vi "Camera_with_init.vi"(0 "Frames":T1=1, 5 "IntegrationTime (us)":dbl=1.0 min=0.1 max=5000.0 step=0.1, 9 "Frame Size (Row x Col)":u16(ring) items=["128x128", "96x128", "64x128", "32x128"], 11 "Timeout":i32) -> (6 "TempK":dbl, 8 "FrameData even":dbl[][][](array[numeric]), 15 "FrameData odd":dbl[][][](array[numeric]))   [LabVIEW 2020]
uses:
  Control 1.ctl
panel:
  out "subarray":dbl[][](array[numeric])
  out "Delta T":dbl[][](array[numeric])
  out "FrameData":dbl[][][](array[numeric])
  out "ExtChData":dbl[][](array[numeric])
  in  "ExChs":i32
  in  "Acq Trigger?":bool
  in  "Offset":i32=128 min=0 max=255 step=1
  out "Actual (us)":dbl
  out "MaxFrameRate":dbl
  out "First Image":dbl[][](graph)
  out "error":errorcluster
  # "IMAGE SETTINGS"
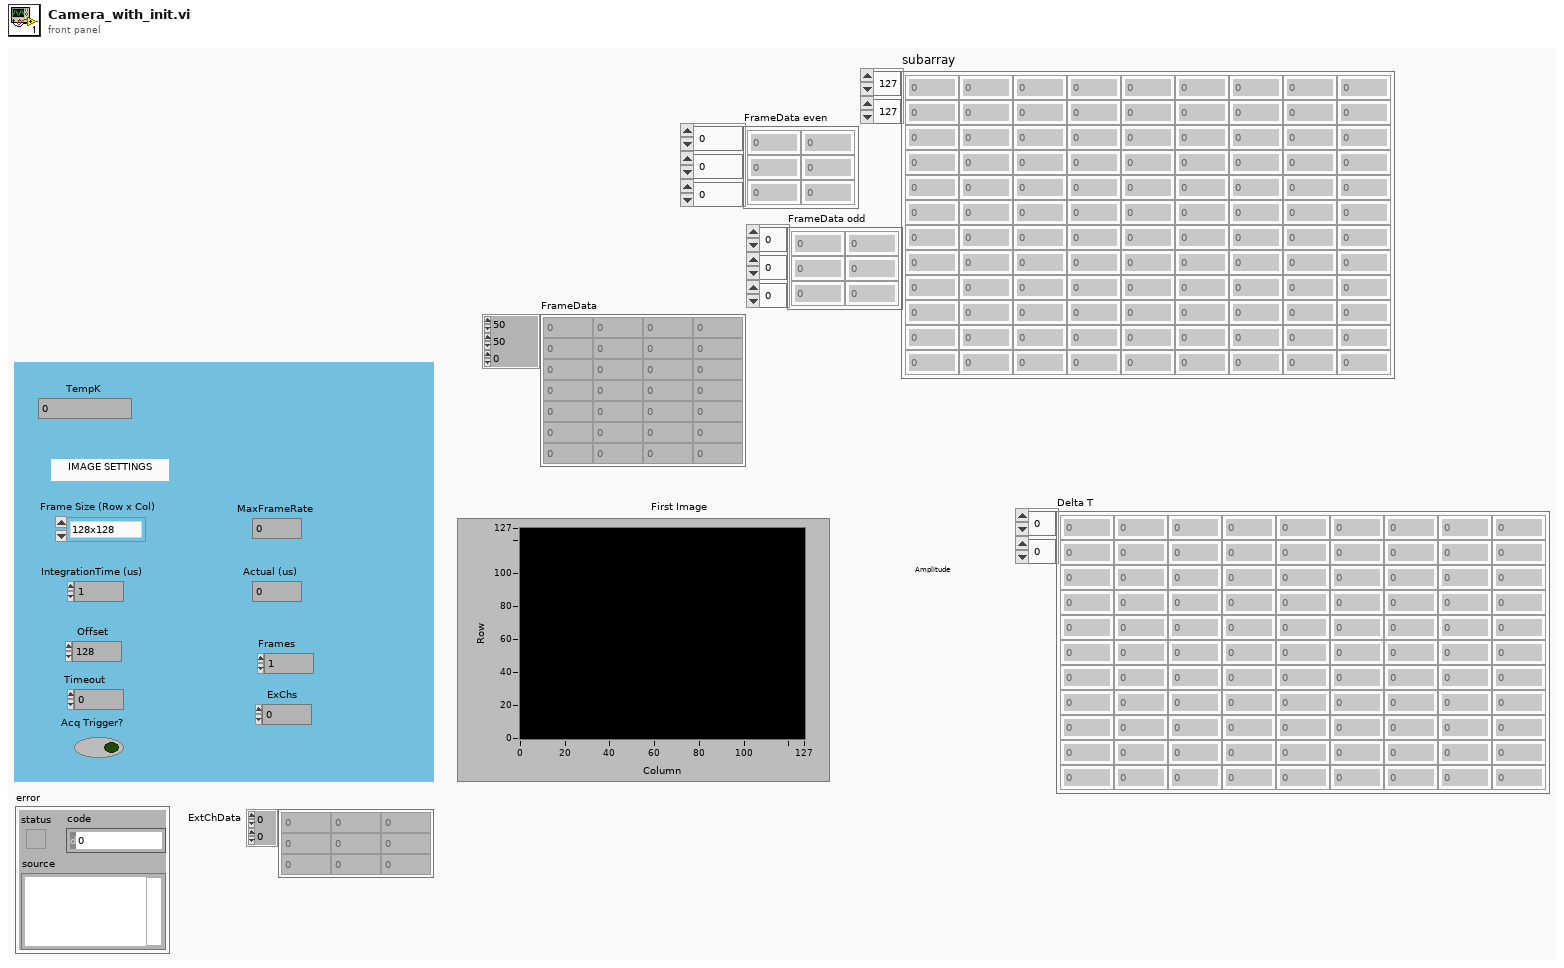
[diagram p1: front panel]
types:
  T1 = typedef "Control 1.ctl" = i32
  T2 = enum16{"big-endian, network order", "native, host order", "little-endian"}
  T3 = enum16{"open", "replace", "create", "open or create", "replace or create", "replace or create with confirmation"}
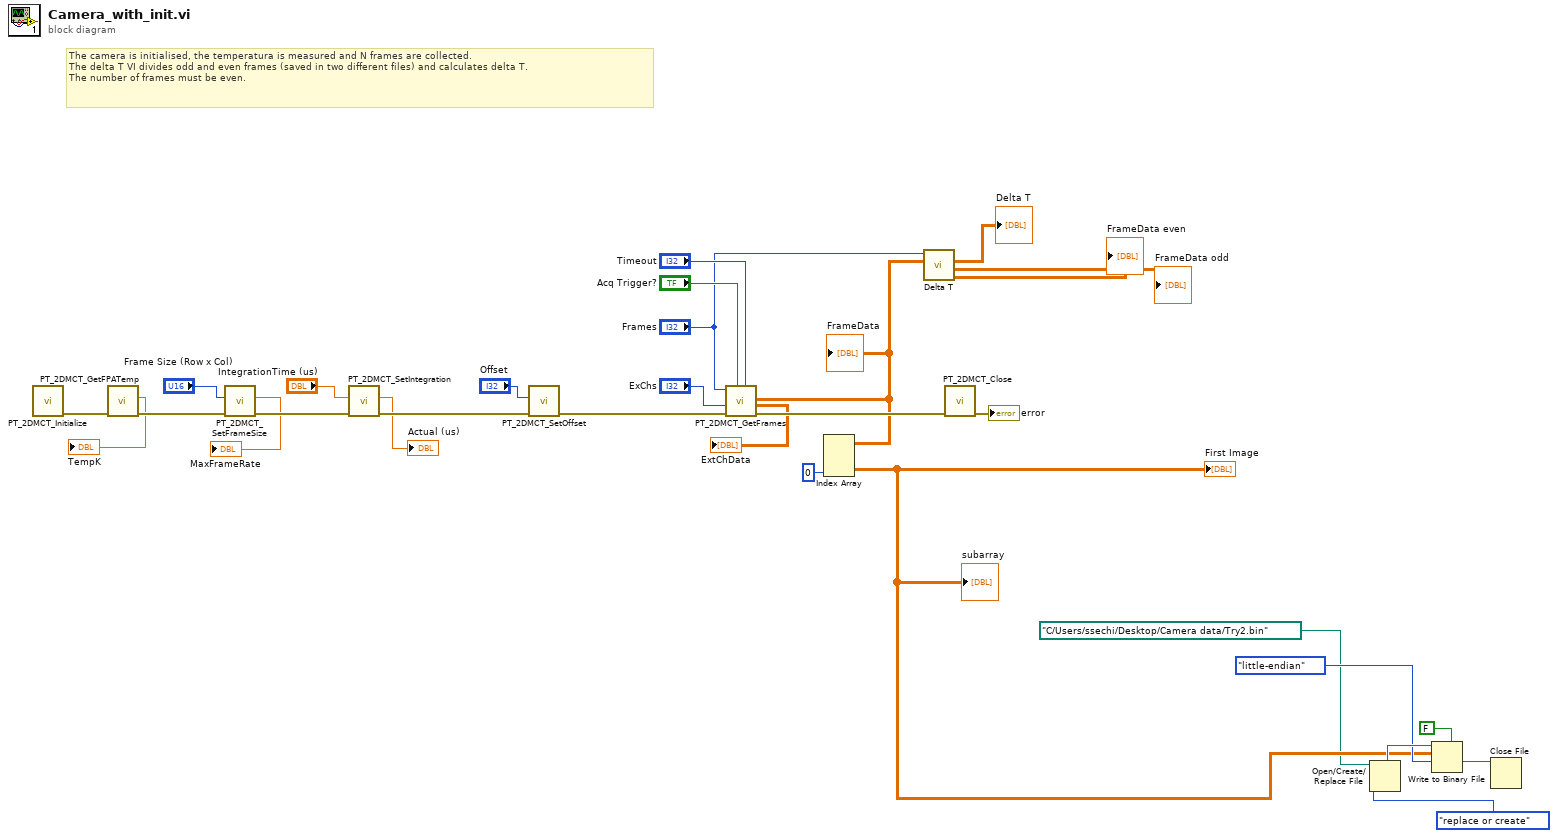
[diagram p0: block diagram]
diagram:
  # "The camera is initialised, the temperatura is measured and N frames are collected. \nThe delta T VI divides odd and even frames (saved in two different files) and calculates delta T.\nThe number of frames must be even."
  n1 = call "PT_2DMCT_Initialize.vi"() -> ("error out"=w27:errorcluster)  [unwired: 11 in]
  n2 = call "PT_2DMCT_GetFPATemp.vi"("error in (no error)"=w27) -> ("error out"=w26:errorcluster, "TempK"=→"TempK":dbl)  [unwired: 8 in, 1 out]
  n3 = call "PT_2DMCT_SetFrameSize.vi"("error in (no error)"=w26, "Frame Size (Row x Col)"="Frame Size (Row x Col)") -> ("error out"=w25:errorcluster, "MaxFrameRate"=→"MaxFrameRate":dbl)  [unwired: 4 in]
  n4 = call "PT_2DMCT_SetIntegration.vi"("error in (no error)"=w25, "IntegrationTime (us)"="IntegrationTime (us)") -> ("error out"=w24:errorcluster, "Actual (us)"=→"Actual (us)":dbl)  [unwired: 4 in]
  n5 = call "PT_2DMCT_SetOffset.vi"("error in (no error)"=w24, "Offset"="Offset") -> ("error out"=w23:errorcluster)  [unwired: 9 in]
  n6 = call "PT_2DMCT_GetFrames.vi"("Timeout"="Timeout", "Acq Trigger?"="Acq Trigger?", "error in (no error)"=w23, "ExChs"="ExChs", "Frames"="Frames") -> ("error out"=w29:errorcluster, "ExtChData"=→"ExtChData":dbl[][], "FrameData"=w8:dbl[][][])  [unwired: 4 in]
  "FrameData" <- w8
  n7 = Index Array(array=w8, index (dim 2)=0 ("disabled index (col)")) -> (element=w2:dbl[][])  [unwired: 2 in]
  "First Image" <- w2
  "subarray" <- w2
  n8 = call "Delta T.vi"("FrameData"=w8, "Number of frames"="Frames") -> ("FrameData even"=→"FrameData even":dbl[][][], "FrameData odd"=→"FrameData odd":dbl[][][], "Delta T"=→"Delta T":dbl[][])  [unwired: 7 in]
  n9 = call "PT_2DMCT_Close.vi"("error in (no error)"=w29) -> ("error out"=→"error":errorcluster)  [unwired: 10 in]
  n10 = Open/Create/Replace File(file path (use dialog)=path "C:/Users/ssechi/Desktop/Camera data/Try2.bin", operation (0:open)=T3."replace or create") -> (refnum out=w7:refnum<file>)  [unwired: 4 in, 2 out]
  n11 = Write to Binary File(file (use dialog)=w7, data=w2, 5:FALSE ("prepend array or string size? (T)"), 9:T2."little-endian" ("byte order (0:big-endian, network order)")) -> (refnum out=w6:refnum<file>)  [unwired: 2 in, 2 out]
  n12 = Close File(refnum=w6) -> ()  [unwired: 1 in, 2 out]
